vi "Validate Hardware.vi"(6 "Interactive":bool, 8 "error in (no error)":errorcluster, 9 "Pane":refnum<vi>, 10 "XY graph ref":refnum<vi>, 11 "Spectrum Recorder in":refnum<class "Spectrum Recorder too.lvclass">) -> (0 "error out":errorcluster, 2 "Valid":bool, 3 "Spectrum Recorder out":refnum<class "Spectrum Recorder too.lvclass">, 4 "Actor's Enqueuer":refnum<class "Message Enqueuer.lvclass">)   [LabVIEW 2016, in "Spectrum Recorder too.lvclass"]
uses:
  Spectrum Recorder too.lvclass
  <vilib>/ActorFramework/Message Enqueuer/Message Enqueuer.lvclass
  Utilities/Cursor Digitizer/Cursor Digitizer.lvclass
  C:/Program Files/National Instruments/LabVIEW 2016/vi.lib/ActorFramework/Actor/Actor.lvclass
  Utilities/Cursor Digitizer/Cursor Digitizer.lvclass/Cursor Digitizer.ctl
  Spectrum Recorder too.lvclass/Spectrum Recorder too.ctl
  Utilities/Cursor Digitizer/Write XY graph ref.vi
  Utilities/Cursor Digitizer/Write Callers pane.vi
  NHMFL_Core/Libraries/Red Pitaya/RP Core/RP Transceiver/RP Transceiver.lvclass
  C:/github/NHMFL_Core/Libraries/Red Pitaya/RP Core/RP Instrument/RP Instrument.lvclass
  Read RP transceiver.vi
  Read Spectrum Recorder Configuration.vi
  NHMFL_Core/Libraries/Red Pitaya/RP Core/RP Instrument/Write Server address.vi
  Write RP transceiver.vi
  <vilib>/ActorFramework/Actor/Actor.lvclass
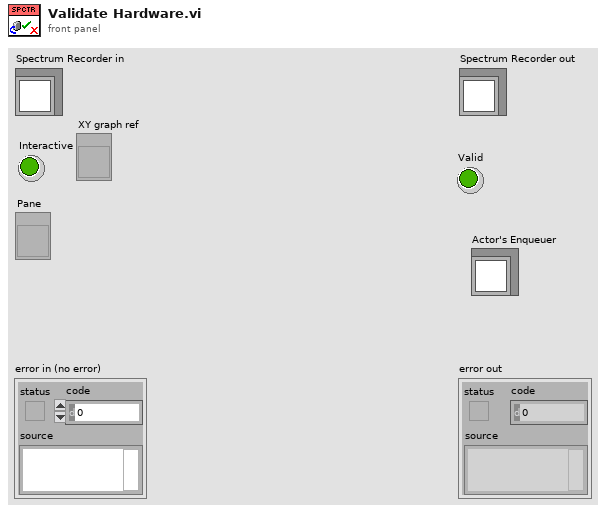
[diagram p1: front panel]
types:
  T1 = typedef "Spectrum Configuration.ctl" = cluster{"Start frequency":dbl, "End frequency":dbl, "Coarse step":dbl, "Step duration":dbl, "Red Pitaya address":string, "Open plot \non start":bool, "Regions width":dbl, "Fine step":dbl, "Pause between scans":dbl, "Clear rgs on start":bool, "Output amplitude":dbl, "Append measurements":string[]}
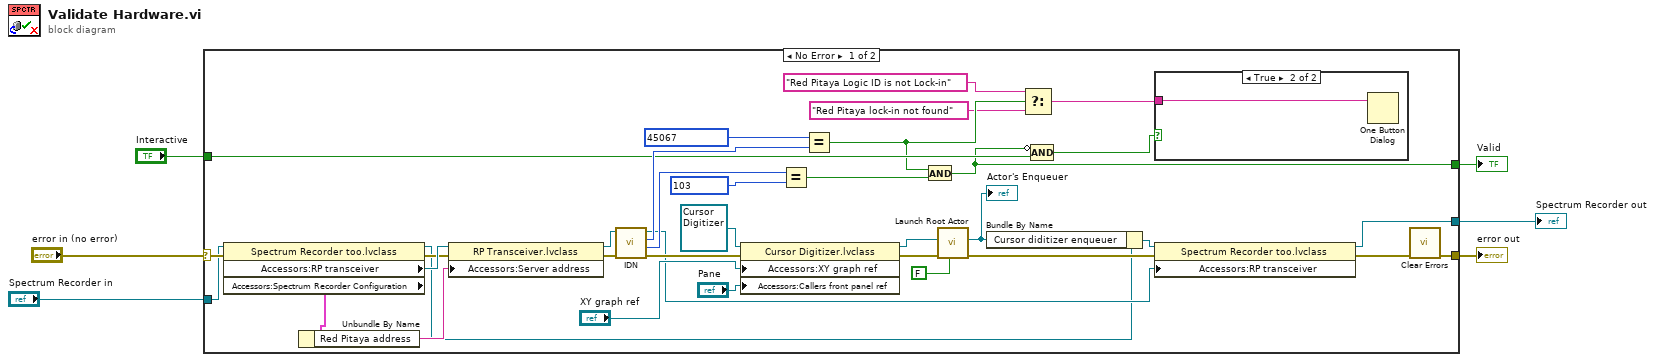
[diagram p0: block diagram]
diagram:
  n1 = case shown="No Error" "error in (no error)" {
    selector: "error in (no error)" -> [w10 w44]
    tunnel: [w34 w44] -> w5
    tunnel: [w15 w43] -> w3
    tunnel: "Spectrum Recorder in" -> [w9 w43]
    tunnel: [w35 _] -> w2
    tunnel: "Interactive" -> [w36 _]
    frame No Error {
      n2 = property class="Spectrum Recorder too.lvclass"(reference=w9, error in=w10) -> (reference out=w8:refnum<class "Spectrum Recorder too.lvclass">, error out=w11:errorcluster, "Accessors:RP transceiver"=w17:refnum<class "RP Transceiver.lvclass">, "Accessors:Spectrum Recorder Configuration"=w7:T1)
      n3 = Unbundle By Name(w7) -> ("Red Pitaya address"=w19:string)
      n4 = property class="RP Transceiver.lvclass"(reference=w17, error in=w11, "Accessors:Server address"=w19) -> (reference out=w20:refnum<class "RP Transceiver.lvclass">, error out=w18:errorcluster)
      n5 = call-dynamic "IDN.vi"("error in (no error)"=w18, "RP Instrument in"=w20) -> ("error out"=w28:errorcluster, "Logic tag"=w38:u16, "IDN response"=w40:u32, "RP Instrument out"=w14:refnum<class "RP Transceiver.lvclass">)  [unwired: 6 in]
      n6 = property class="Cursor Digitizer.lvclass"(reference=refnum<class "Cursor Digitizer.lvclass"> refnum ("Cursor Digitizer.lvclass"), error in=w28, "Accessors:XY graph ref"="XY graph ref", "Accessors:Callers front panel ref"="Pane") -> (reference out=w23:refnum<class "Cursor Digitizer.lvclass">, error out=w25:errorcluster)
      n7 = Equal?(x=w38, y=u16 103 ("IDN response")) -> (x = y?=w37:bool)
      n8 = Equal?(x=u32 45067 ("IDN response"), y=w40) -> (x = y?=w32:bool)
      n9 = And(x=w32, y=w37) -> (x .and. y?=w35:bool)
      n10 = call <vilib>:"Launch Root Actor.vi"("Open Actor Core front panel? (F)"=FALSE, "error in (no error)"=w25, "Actor"=w23) -> ("error out"=w13:errorcluster, "Actor's Enqueuer"=w26:refnum<class "Message Enqueuer.lvclass">)  [unwired: 7 in]
      "Actor's Enqueuer" <- w26
      n11 = Bundle By Name(cluster=w8, "Cursor diditizer enqueuer"=w26) -> (w16:refnum<class "Spectrum Recorder too.lvclass">)
      n12 = Select(t="Red Pitaya Logic ID is not Lock-in" ("message"), s=w32, f="Red Pitaya lock-in not found" ("message")) -> (s? t:f=w29:string)
      n13 = Compound Arithmetic op=AND(invert w35, w36) -> (w33:bool)
      n14 = case shown="True" w33 {
        tunnel: w29 -> [_ w42]
        frame False {
        }
        frame True {
          n15 = One Button Dialog(message=w42) -> ()  [unwired: 1 in, 1 out]
        }
      }
      n16 = property class="Spectrum Recorder too.lvclass"(reference=w16, error in=w13, "Accessors:RP transceiver"=w14) -> (reference out=w15:refnum<class "Spectrum Recorder too.lvclass">, error out=w12:errorcluster)
      n17 = call <vilib>:"Clear Errors.vi"("error in (no error)"=w12) -> ("error out"=w34:errorcluster)  [unwired: 5 in, 1 out]
    }
    frame Error {
    }
  }
  "error out" <- w5
  "Spectrum Recorder out" <- w3
  "Valid" <- w2
